vi "GuessRandomNumbers.vi"() -> ()   [LabVIEW 2019]
uses:
  <vilib>/numeric/Random Number (Range) U64.vi
panel:
  out "System Guess":i32
  out "you Win or Not":bool
  in  "Guess Number":dbl
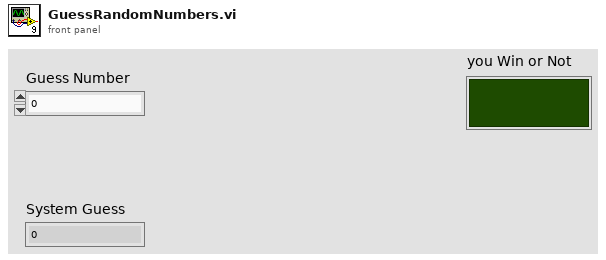
[diagram p1: front panel]
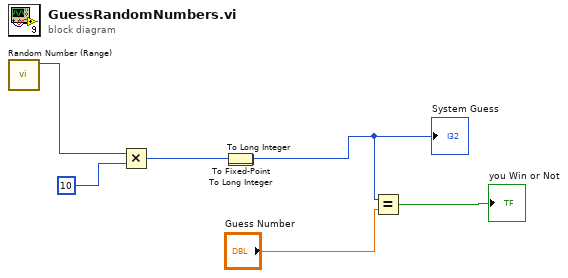
[diagram p0: block diagram]
diagram:
  n1 = call-poly <vilib>:"Random Number (Range).vi"() -> ("number"=w6:u64)  [unwired: 11 in]
  n2 = Multiply(x=w6, y=u64 10) -> (x*y=w4:u64)
  n3 = To Long Integer(number=w4) -> (32bit integer=w3:i32)
  "System Guess" <- w3
  n4 = To Long Integer() -> ()  [unwired: 1 in, 1 out]
  n5 = To Fixed-Point() -> ()  [unwired: 2 in, 1 out]
  n6 = Equal?(x=w3, y="Guess Number") -> (x = y?=→"you Win or Not":bool)
